vi "Parse Brass ERD.vi"(0 "string":string) -> (14 "Folding":i32, 16 "Jerk":i32)   [LabVIEW 2016]
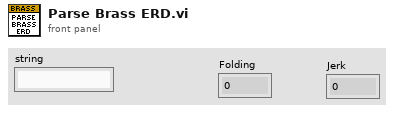
[diagram p1: front panel]
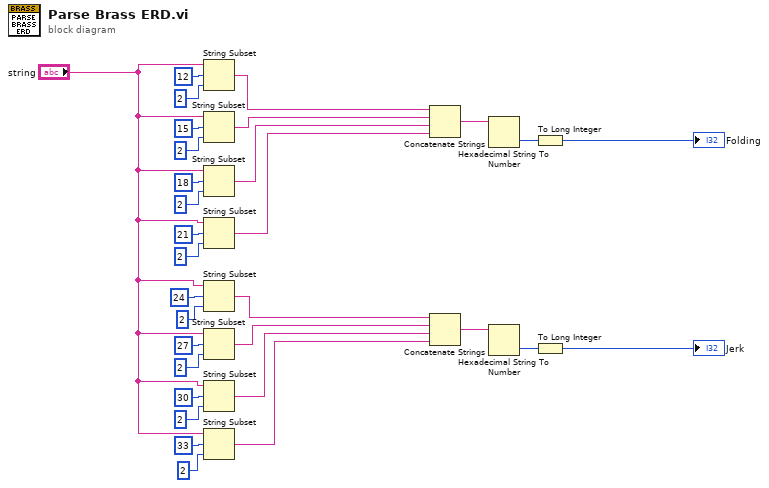
[diagram p0: block diagram]
diagram:
  n1 = String Subset(string="string", offset (0)=12, length (rest)=2 ("length (rest)")) -> (substring=w12:string)
  n2 = String Subset(string="string", offset (0)=15, length (rest)=2 ("length (rest)")) -> (substring=w11:string)
  n3 = String Subset(string="string", offset (0)=18, length (rest)=2 ("length (rest)")) -> (substring=w10:string)
  n4 = String Subset(string="string", offset (0)=21, length (rest)=2 ("length (rest)")) -> (substring=w9:string)
  n5 = String Subset(string="string", offset (0)=24, length (rest)=2 ("length (rest)")) -> (substring=w5:string)
  n6 = String Subset(string="string", offset (0)=27, length (rest)=2 ("length (rest)")) -> (substring=w4:string)
  n7 = String Subset(string="string", offset (0)=30, length (rest)=2 ("length (rest)")) -> (substring=w3:string)
  n8 = String Subset(string="string", offset (0)=33, length (rest)=2 ("length (rest)")) -> (substring=w2:string)
  n9 = Concatenate Strings(w12, w11, w10, w9) -> (w13:string)
  n10 = Concatenate Strings(w5, w4, w3, w2) -> (w7:string)
  n11 = Hexadecimal String To Number(string=w13) -> (number=w14:u32)  [unwired: 2 in, 1 out]
  n12 = Hexadecimal String To Number(string=w7) -> (number=w6:u32)  [unwired: 2 in, 1 out]
  n13 = To Long Integer(number=w14) -> (32bit integer=→"Folding":i32)
  n14 = To Long Integer(number=w6) -> (32bit integer=→"Jerk":i32)
